vi "Release Queue.vi"(8 "error in":errorcluster, 11 "QueueMessageTransport in":refnum<class "QueueMessageTransport.lvclass">) -> (0 "error out":errorcluster, 3 "QueueMessageTransport out":refnum<class "QueueMessageTransport.lvclass">)   [LabVIEW 2016, in "QueueMessageTransport.lvclass"]
doc: "This public method releases a reference to the Queue\n\n\nAuthor: Stas Legedza"
uses:
  QueueMessageTransport.lvclass
  QueueMessageTransport.lvclass/QueueMessageTransport.ctl
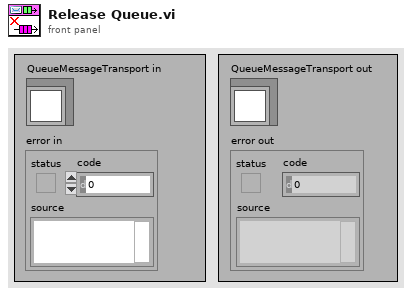
[diagram p1: front panel]
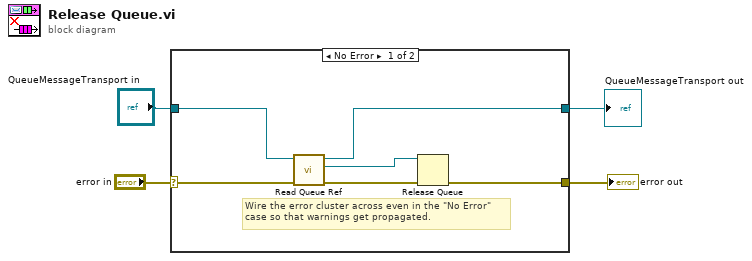
[diagram p0: block diagram]
diagram:
  n1 = case shown="No Error" "error in" {
    selector: "error in" -> [w10 w12]
    tunnel: [w5 w12] -> w3
    tunnel: [w6 w11] -> w1
    tunnel: "QueueMessageTransport in" -> [w7 w11]
    frame No Error {
      # "Wire the error cluster across even in the \"No Error\"\ncase so that warnings get propagated."
      n2 = call "Read Queue Ref.vi"("error in"=w10, "QueueMessageTransport in"=w7) -> ("error out"=w9:errorcluster, "Queue Ref"=w8:refnum<queue>, "QueueMessageTransport out"=w6:refnum<class "QueueMessageTransport.lvclass">)  [unwired: 7 in]
      n3 = Release Queue(queue=w8, error in (no error)=w9) -> (error out=w5:errorcluster)  [unwired: 1 in, 2 out]
    }
    frame Error {
    }
  }
  "error out" <- w3
  "QueueMessageTransport out" <- w1
